vi "ValueChange.vi"(8 "error in (no error)":errorcluster, 11 "Calendar in":refnum<class "Calendar.lvclass">) -> (0 "error out":errorcluster, 3 "Calendar out":refnum<class "Calendar.lvclass">)   [LabVIEW 2015, in "Calendar.lvclass"]
uses:
  Calendar.lvclass
  Calendar.lvclass/Calendar.ctl
  Read CalendarValue.vi
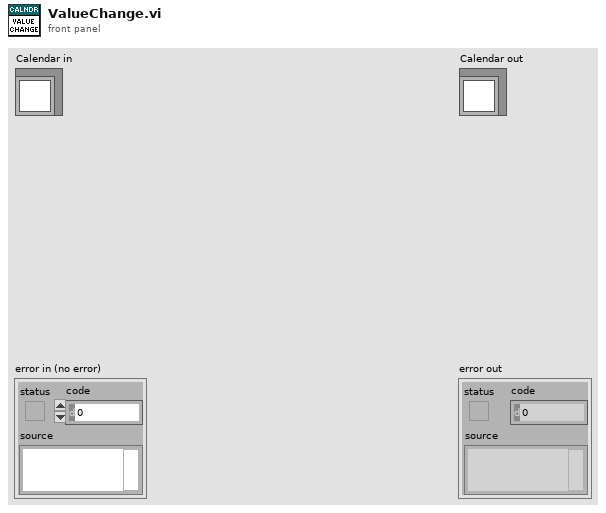
[diagram p1: front panel]
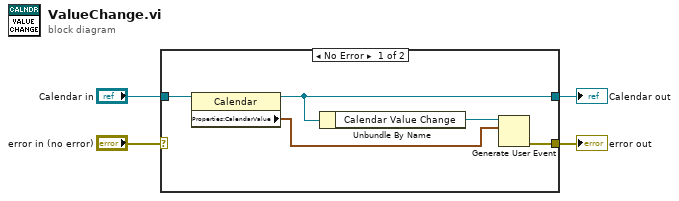
[diagram p0: block diagram]
diagram:
  n1 = case shown="No Error" "error in (no error)" {
    selector: "error in (no error)" -> [_ w11]
    tunnel: [w5 w11] -> w3
    tunnel: [w8 w10] -> w1
    tunnel: "Calendar in" -> [w9 w10]
    frame No Error {
      n2 = property class="Calendar"(reference=w9) -> (reference out=w8:refnum<class "Calendar.lvclass">, "Properties:CalendarValue"=w6:timestamp)  [unwired: 1 in, 1 out]
      n3 = Unbundle By Name(w8) -> ("Calendar Value Change"=w7:refnum<user-event>)
      n4 = Generate User Event(user event=w7, event data cluster=w6) -> (error out=w5:errorcluster)  [unwired: 2 in, 1 out]
    }
    frame Error {
    }
  }
  "error out" <- w3
  "Calendar out" <- w1
